vi "From String Tree Data.vi"(11 "Tree Data":refnum<class "Tree Data.lvclass">) -> (2 "String":string)   [LabVIEW 2017, in "Tree API.lvlib" / "String.lvclass"]
doc: "Extract a String value from Tree Data type."
uses:
  String.lvclass
  Tree Data/Tree Data.lvclass
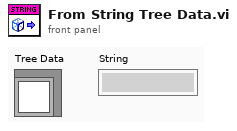
[diagram p1: front panel]
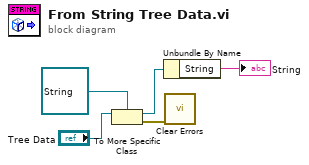
[diagram p0: block diagram]
diagram:
  n1 = To More Specific Class(target class=refnum<class "String.lvclass"> refnum ("String.lvclass"), reference="Tree Data") -> (specific class reference=w1:refnum<class "String.lvclass">, error out=w2:errorcluster)  [unwired: 1 in]
  n2 = Unbundle By Name(w1) -> ("String"=→"String":string)
  n3 = call <vilib>:"Clear Errors.vi"("error in (no error)"=w2) -> ()  [unwired: 5 in, 2 out]
